vi "Day 14-Add to Letter Count.vi"(9 "Count":u64, 10 "New Entry":u8, 11 "Count Array in":u64[](array[numeric])) -> (3 "Count Array out":u64[](array[numeric]))   [LabVIEW 2021]
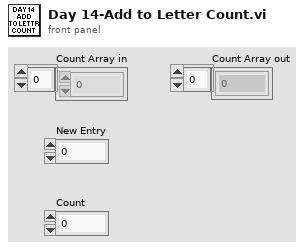
[diagram p1: front panel]
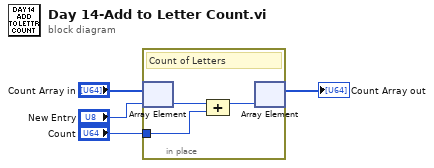
[diagram p0: block diagram]
diagram:
  n1 = in-place {
    in-place-border: "Count" -> [w7]
    # "Count of Letters"
    n2 = in-place-array #1("Count Array in", "New Entry") -> (w6:u64)
    n3 = Compound Arithmetic op=ADD(w6, w7) -> (w5:u64)
    n4 = in-place-array #1(w5) -> (→"Count Array out":u64[])  [unwired: 1 out]
  }
